vi "get_input.vi"(8 "error in (no error)":errorcluster, 11 "input_poller in":refnum<class "input_poller.lvclass">) -> (0 "error out":errorcluster, 2 "input":i32, 3 "input_poller out":refnum<class "input_poller.lvclass">)   [LabVIEW 2015, in "input_poller.lvclass"]
uses:
  input_poller.lvclass
  input_poller.lvclass/input_poller.ctl
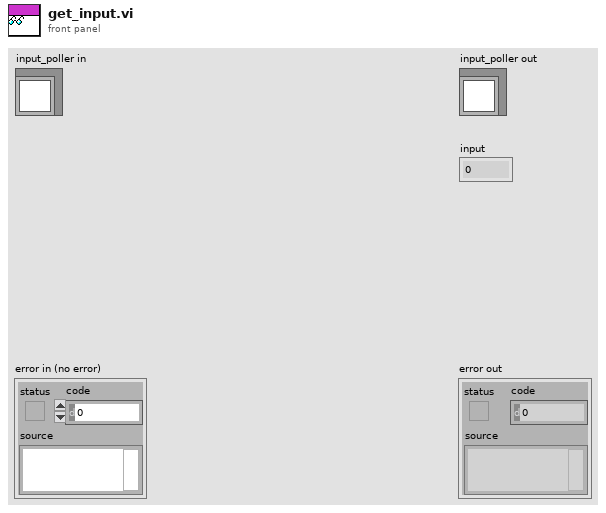
[diagram p1: front panel]
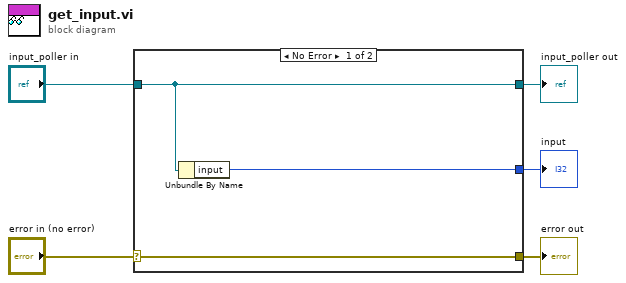
[diagram p0: block diagram]
diagram:
  n1 = case shown="No Error" "error in (no error)" {
    selector: "error in (no error)" -> [w8 w9]
    tunnel: [w8 w9] -> w4
    tunnel: [w7 w10] -> w2
    tunnel: "input_poller in" -> [w7 w10]
    tunnel: [w6 _] -> w1
    frame No Error {
      n2 = Unbundle By Name(w7) -> ("input"=w6:i32)
    }
    frame Error {
    }
  }
  "error out" <- w4
  "input_poller out" <- w2
  "input" <- w1
